vi "Fasor.vi"() -> ()   [LabVIEW 2015]
panel:
  in  "data array [mag, phase (deg)]":cluster{"magnitude":dbl, "phase":dbl}[](array[cluster]) {"phase" format="%0.2f"; "magnitude" format="%0.2f"}
  out "Polar Plot":picture
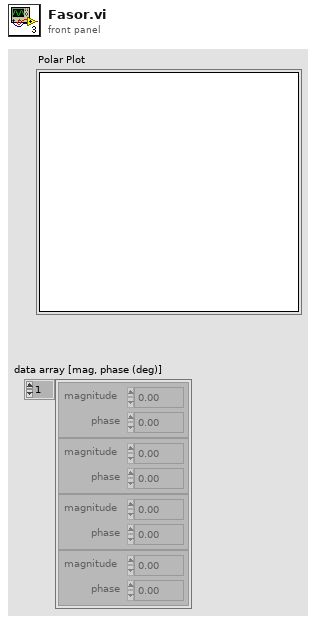
[diagram p1: front panel]
types:
  T1 = typedef "LVBoundsTypeDef.ctl" = cluster{"Width":u32, "Height":u32}
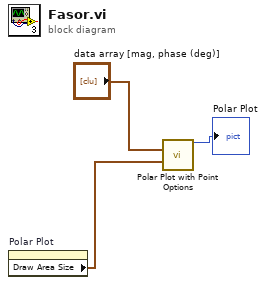
[diagram p0: block diagram]
diagram:
  n1 = property on="Polar Plot" class="Pict"() -> ("Draw Area Size"=w2:T1)  [unwired: 2 in, 2 out]
  n2 = call <vilib>:"Polar Plot with Point Options.vi"("data array [mag, phase (deg)]"="data array [mag, phase (deg)]", "dimensions (w,h)"=w2) -> ("new picture"=→"Polar Plot":picture)  [unwired: 13 in]
